vi "Get Images.vi"(0 "first":i32, 1 "validfirst":i32, 5 "last":i32, 7 "arr":i32, 9 "size":u32, 11 "error in (no error)":errorcluster, 12 "validlast":i32) -> (3 "validfirst out":i32, 4 "function return":u32, 8 "arr out":i32, 14 "validlast out":i32, 15 "error out":errorcluster)   [LabVIEW 2014, in "atmcd32d.lvlib"]
doc: "unsigned int WINAPI GetImages(long first, long last, at_32 * arr, unsigned long size, long * validfirst, long * validlast);"
uses:
  atmcd32d.lvlib
  atmcd32d.dll
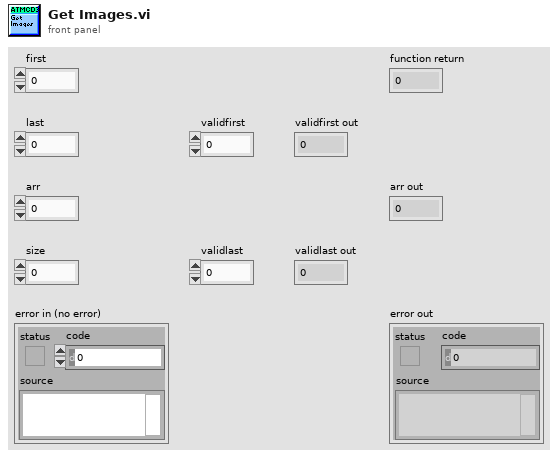
[diagram p1: front panel]
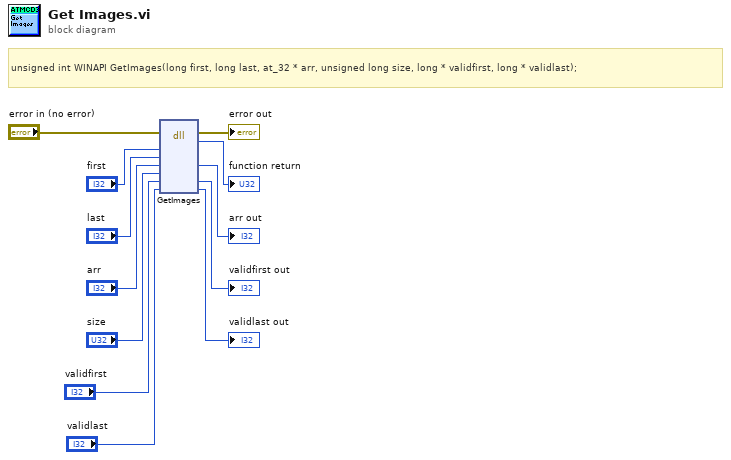
[diagram p0: block diagram]
diagram:
  # "unsigned int WINAPI GetImages(long first, long last, at_32 * arr, unsigned long size, long * validfirst, long * validlast);"
  n1 = dll-call lib="C:/Users/Bakir/Documents/Lambda2-Testing/lib/Andorlib/atmcd32d.*" fn="GetImages"(error in="error in (no error)", "first"="first", "last"="last", "arr"="arr", "size"="size", "validfirst"="validfirst", "validlast"="validlast") -> (error out=→"error out":errorcluster, →"function return":u32, "arr"=→"arr out":i32, "validfirst"=→"validfirst out":i32, "validlast"=→"validlast out":i32)  [unwired: 5 in, 1 out]
